vi "Do Request.vi"(7 "Processing In":refnum<class "Processing.lvclass">, 11 "InfoController in":refnum<class "InfoController.lvclass">) -> (0 "error out":errorcluster, 5 "Processing":refnum<class "Processing.lvclass">)   [LabVIEW 2020, in "Vecto.lvlib" / "InfoController.lvclass"]
uses:
  InfoController.lvclass
  <vilib>/IlluminatedG/IG HTTP Server/HTTP Server/Processing/Processing.lvclass
  Info Segment.ctl
  <vilib>/IlluminatedG/IG HTTP Server/HTTP Server/Processing/Processing.lvclass/Processing.ctl
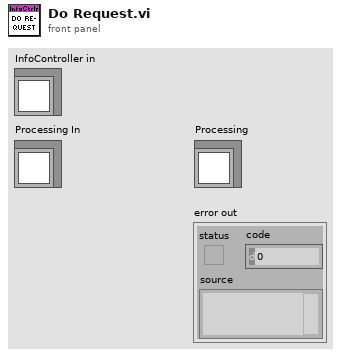
[diagram p1: front panel]
types:
  T1 = typedef "Vecto.lvlib/InfoController.lvclass/Info Segment.ctl" = enum16{"UNKNOWN", "node", "status", "health"}
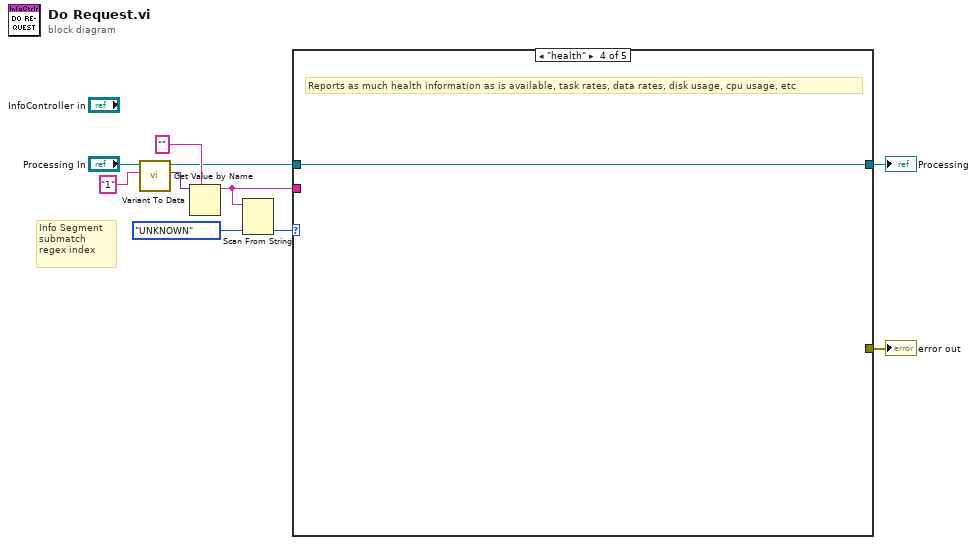
[diagram p0: block diagram]
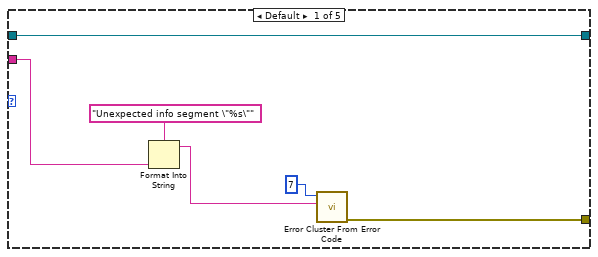
[diagram p2: hidden frame]
diagram:
  # "Info Segment submatch regex index"
  n1 = call <vilib>:"Get Value by Name.vi"("Name"="1", "Processing in"="Processing In") -> ("Value"=w8:variant, "Processing out"=w6:refnum<class "Processing.lvclass">)  [unwired: 7 in, 1 out]
  n2 = Variant To Data(type="", Variant=w8) -> (data=w3:string)  [unwired: 1 in, 1 out]
  n3 = Scan From String(input string=w3, default 1=Info_Segment."UNKNOWN" ("Info Segment")) -> (output 1=w4:T1)  [unwired: 3 in, 3 out]
  n4 = case shown="\"health\"" w4 {
    tunnel: w6 -> [w11 w17 w18 w19 w20]
    tunnel: w3 -> [w14 _ _ _ _]
    tunnel: [w12 _ _ _ _] -> w2
    tunnel: [w11 w17 w18 w19 w20] -> w1
    frame Default {
      n5 = Format Into String(format string="Unexpected info segment \"%s\"", w14) -> (resulting string=w13:string)  [unwired: 2 in, 1 out]
      n6 = call <vilib>:"Error Cluster From Error Code.vi"("error message (\"\")"=w13, "error code (0)"=7) -> ("error out"=w12:errorcluster)  [unwired: 7 in]
    }
    frame "node" {
      # "Return node info"
    }
    frame "status" {
      # "Vecto connection and node status"
    }
    frame "health" {
      # "Reports as much health information as is available, task rates, data rates, disk usage, cpu usage, etc"
    }
    frame "UNKNOWN" {
    }
  }
  "error out" <- w2
  "Processing" <- w1
